vi "solar_ui Resize.vi"(8 "error in (no error)":errorcluster, 9 "Panes":T1={"Status"=TRUE, "Emergency"=TRUE, "Targets"=TRUE}, 10 "MenuRef":refnum<k9>, 11 "VI Refnum":refnum<vi>) -> (0 "error out":errorcluster)   [LabVIEW 2018]
doc: "This resizes the panes of the SOLAR user interface depending on which pane is visible. If the Targets pane is hidden, the emergency stop is hidden as well."
uses:
  <vilib>/Utility/miscctls.llb/LVPointTypeDef.ctl
  solar_ctl SOLAR UI Panes.ctl
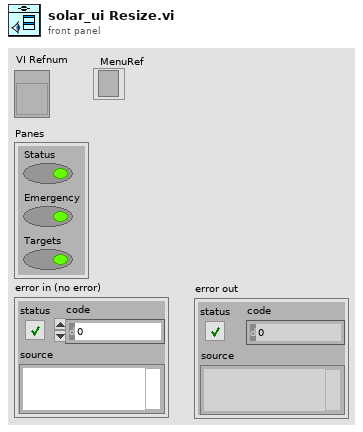
[diagram p1: front panel]
types:
  T1 = typedef "solar_ctl SOLAR UI Panes.ctl" = cluster{"Status":bool, "Emergency":bool, "Targets":bool}
  T2 = enum16{"No Scaling", "Scale All Objects", "Scale Single Object"}
  T3 = typedef "LVBoundsTypeDef.ctl" = cluster{"Width":u32, "Height":u32}
  T4 = typedef "LVMenuShortCut.ctl" = cluster{"include Shift key?":bool, "include Ctrl key?":bool, "shortcut key":string}
  T5 = enum16{"No Scaling", "Scale All Objects", "Scale Single Object"}[]
  T6 = typedef "LVPointTypeDef.ctl" = cluster{"Horizontal":i16, "Vertical":i16}
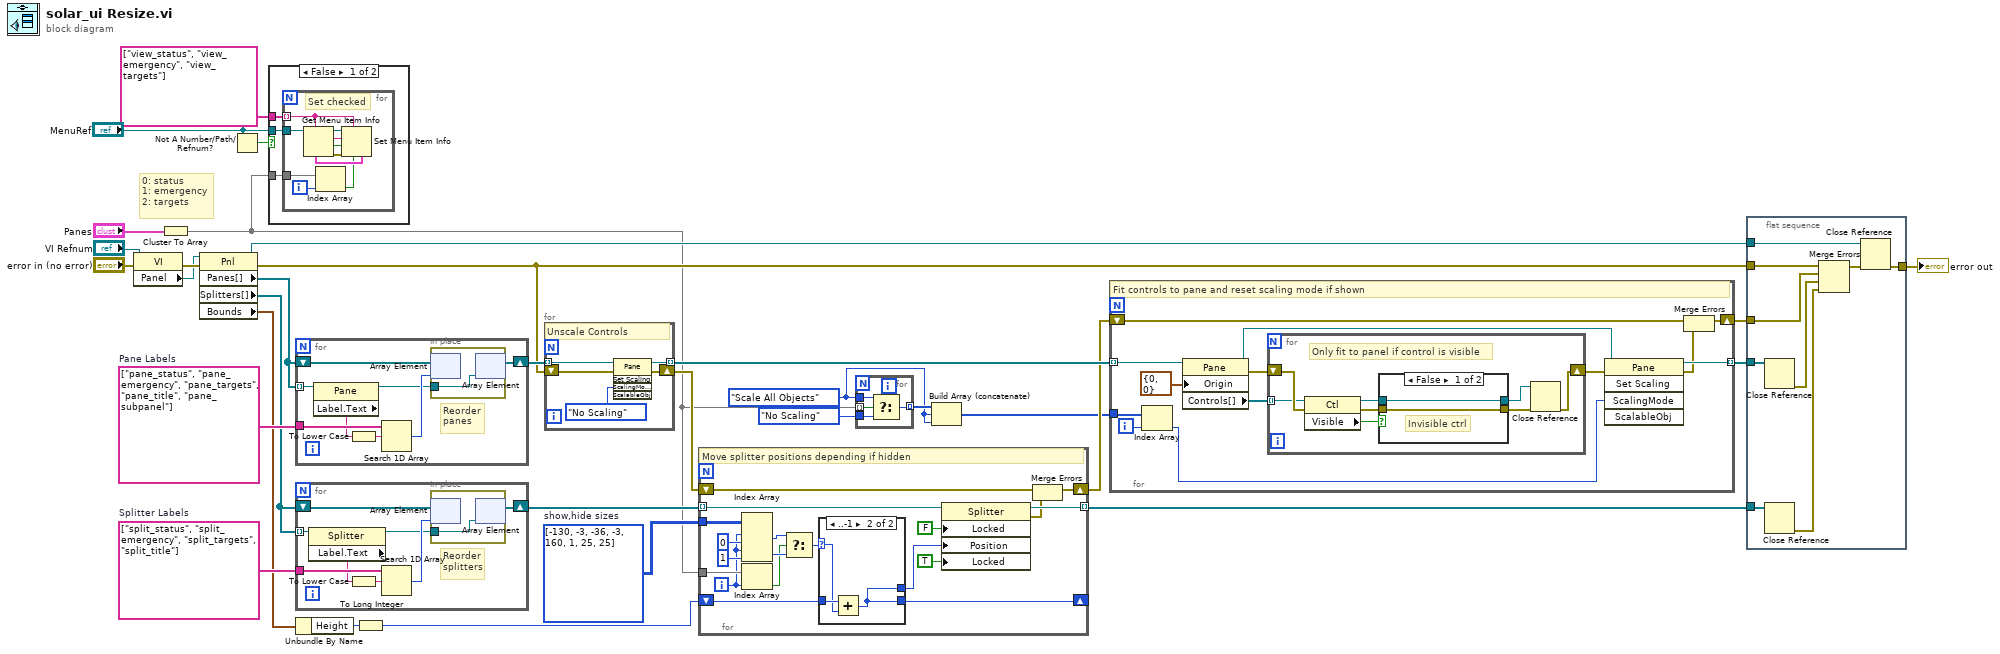
[diagram p0: block diagram]
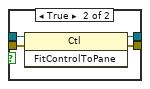
[diagram p3: hidden frame]
diagram:
  w10 = T2."Scale All Objects" ("Scaling Mode")
  w14 = i32[][] [[-130, -3], [-36, -3], [160, 1], [25, 25]]  # show,hide sizes
  w26 = string[] ["split_status", "split_emergency", "split_targets", "split_title"]  # Splitter Labels
  w28 = string[] ["pane_status", "pane_emergency", "pane_targets", "pane_title", "pane_subpanel"]  # Pane Labels
  # "0: status\n1: emergency\n2: targets"
  n1 = property class="VI"(reference="VI Refnum", error in="error in (no error)") -> (error out=w30:errorcluster, "Panel"=w29:refnum<vi>)  [unwired: 1 out]
  n2 = Cluster To Array(cluster="Panes") -> (array=w1:bool[])
  n3 = property class="Pnl"(reference=w29, error in=w30) -> (reference out=w7:refnum<vi>, error out=w21:errorcluster, "Panes[]"=w27:refnum<vi>[], "Splitters[]"=w25:refnum<vi>[], "Bounds"=w3:T3)
  n4 = Not A Number/Path/Refnum?(number/path/refnum="MenuRef") -> (NaN/Path/Refnum?=w4:bool)
  n5 = case shown="False" w4 {
    tunnel: string[] ["view_status", "view_emergency", "view_targets"] -> [w34 _]
    tunnel: "MenuRef" -> [w35 _]
    tunnel: w1 -> [w33 _]
    frame False {
      n6 = for {
        tunnel: w35 -> [w41]
        tunnel: w33 -> [w39]
        tunnel: w34 -> [w36] mode=indexing
        i -> [w38]
        # "Set checked"
        n7 = Get Menu Item Info(7:w36, 11:w41) -> (0:w45:errorcluster, 1:w42:bool, 2:w43:string, 3:w44:refnum<k9>, 6:w40:T4)  [unwired: 1 in, 2 out]
        n8 = Index Array(array=w39, index=w38) -> (element=w37:bool)
        n9 = Set Menu Item Info(4:w40, 6:w37, 7:w36, 8:w45, 9:w42, 10:w43, 11:w44) -> ()  [unwired: 2 out]
      }
    }
    frame True {
    }
  }
  n10 = for {
    tunnel: w27 -> [w53] mode=indexing
    tunnel: w28 -> [w52]
    shift-right: [w46] -> w22
    shift-left: w27 -> [w49]
    # "Reorder\npanes"
    n11 = property class="Pane"(reference=w53) -> (reference out=w47:refnum<vi>, "Label.Text"=w51:string)  [unwired: 1 in, 1 out]
    n12 = To Lower Case(string=w51) -> (all lower case string=w50:string)
    n13 = Search 1D Array(1D array=w52, element=w50) -> (index of element=w48:i32)  [unwired: 1 in]
    n14 = in-place {
      in-place-border: w47 -> [w54]
      n15 = in-place-array #1(w49, w48) -> ()  [unwired: 1 out]
      n16 = in-place-array #1(w54) -> (w46:refnum<vi>[])  [unwired: 1 out]
    }
  }
  n17 = for {
    tunnel: w25 -> [w62] mode=indexing
    tunnel: w26 -> [w61]
    shift-right: [w55] -> w24
    shift-left: w25 -> [w58]
    # "Reorder\nsplitters"
    n18 = property class="Splitter"(reference=w62) -> (reference out=w56:refnum<vi>, "Label.Text"=w60:string)  [unwired: 1 in, 1 out]
    n19 = To Lower Case(string=w60) -> (all lower case string=w59:string)
    n20 = Search 1D Array(1D array=w61, element=w59) -> (index of element=w57:i32)  [unwired: 1 in]
    n21 = in-place {
      in-place-border: w56 -> [w63]
      n22 = in-place-array #2(w58, w57) -> ()  [unwired: 1 out]
      n23 = in-place-array #2(w63) -> (w55:refnum<vi>[])  [unwired: 1 out]
    }
  }
  n24 = Unbundle By Name(w3) -> ("Height"=w13:u32)
  n25 = To Long Integer(number=w13) -> (32bit integer=w8:i32)
  n26 = for {
    tunnel: w22 -> [w68] mode=indexing
    tunnel: [w64] -> w18 mode=indexing
    shift-right: [w65] -> w20
    shift-left: w21 -> [w66]
    # "Unscale Controls"
    n27 = invoke class="Pane" method="Set Scaling"(reference=w68, error in=w66, "ScalingMode"=T2."No Scaling" ("Scaling Mode")) -> (reference out=w64:refnum<vi>, error out=w65:errorcluster)  [unwired: 2 in, 3 out]
  }
  n28 = for {
    tunnel: w24 -> [w87] mode=indexing
    tunnel: [w85] -> w17 mode=indexing
    shift-right: [w72] -> w16
    shift-left: w20 -> [w71]
    tunnel: w14 -> [w83]
    tunnel: w1 -> [w82]
    shift-right: [w77] -> _
    shift-left: w8 -> [w78]
    i -> [w73]
    # "Move splitter positions depending if hidden"
    n29 = Index Array(array=w83, index (row) #1=w73, index (col) #1=0 ("disabled index (col)"), index (row) #2=w73, index (col) #2=1 ("disabled index (col)")) -> (element #1=w80:i32, element #2=w81:i32)
    n30 = Index Array(array=w82, index=w73) -> (element=w74:bool)
    n31 = Select(t=w80, s=w74, f=w81) -> (s? t:f=w79:i32)
    n32 = case shown="..-1" w79 {
      selector: w79 -> [w88 w90]
      tunnel: w78 -> [w89 w92]
      tunnel: [w89 w91] -> w77
      tunnel: [w88 w91] -> w69
      frame 0.. {
      }
      frame ..-1 {
        n33 = Add(x=w92, y=w90) -> (x+y=w91:i32)
      }
    }
    n34 = property class="Splitter"(reference=w87, "Locked"=FALSE ("Splitter Position Locked"), "Position"=w69, "Locked"=TRUE ("Splitter Position Locked")) -> (reference out=w85:refnum<vi>, error out=w70:errorcluster)  [unwired: 1 in]
    n35 = Merge Errors(w71, w70) -> (w72:errorcluster)
  }
  n36 = for {
    tunnel: w1 -> [w96] mode=indexing
    tunnel: w10 -> [w95]
    tunnel: T2."No Scaling" ("Scaling Mode") -> [w94]
    tunnel: [w93] -> w11 mode=indexing
    n37 = Select(t=w95, s=w96, f=w94) -> (s? t:f=w93:T2)
  }
  n38 = Build Array (concatenate)(w11, w10, w10) -> (w9:T5)
  n39 = for {
    tunnel: w18 -> [w109] mode=indexing
    tunnel: [w108] -> w19 mode=indexing
    shift-right: [w104] -> w15
    shift-left: w16 -> [w105]
    tunnel: w9 -> [w106]
    i -> [w107]
    # "Fit controls to pane and reset scaling mode if shown"
    n40 = Index Array(array=w106, index=w107) -> (element=w97:T2)
    n41 = property class="Pane"(reference=w109, "Origin"=T6 {"Horizontal"=0, "Vertical"=0}) -> (reference out=w102:refnum<vi>, error out=w100:errorcluster, "Controls[]"=w98:refnum<vi>[])  [unwired: 1 in]
    n42 = for {
      tunnel: w98 -> [w112] mode=indexing
      shift-right: [w115] -> w99
      shift-left: w100 -> [w117]
      # "Only fit to panel if control is visible"
      n43 = property class="Ctl"(reference=w112, error in=w117) -> (reference out=w111:refnum<vi>, error out=w113:errorcluster, "Visible"=w110:bool)
      n44 = case shown="False" w110 {
        tunnel: [w119 w123] -> w116
        tunnel: [w118 w122] -> w114
        tunnel: w113 -> [w119 w121]
        tunnel: w111 -> [w118 w120]
        frame False {
          # "Invisible ctrl"
        }
        frame True {
          n45 = invoke class="Ctl" method="FitControlToPane"(reference=w120, error in=w121) -> (reference out=w122:refnum<vi>, error out=w123:errorcluster)  [unwired: 1 in, 1 out]
        }
      }
      n46 = Close Reference(reference=w114, error in (no error)=w116) -> (error out=w115:errorcluster)
    }
    n47 = invoke class="Pane" method="Set Scaling"(reference=w102, error in=w99, "ScalingMode"=w97) -> (reference out=w108:refnum<vi>, error out=w103:errorcluster)  [unwired: 2 in, 3 out]
    n48 = Merge Errors(w105, w103) -> (w104:errorcluster)
  }
  n49 = flat-sequence {
    tunnel: [w129] -> w23
    tunnel: w7 -> [w128]
    tunnel: w21 -> [w127]
    tunnel: w19 -> [w126]
    tunnel: w17 -> [w125]
    tunnel: w15 -> [w124]
    frame #0 {
      n50 = Close Reference(reference=w126) -> (error out=w131:errorcluster)  [unwired: 1 in]
      n51 = Close Reference(reference=w125) -> (error out=w130:errorcluster)  [unwired: 1 in]
      n52 = Merge Errors(w127, w124, w131, w130) -> (w132:errorcluster)
      n53 = Close Reference(reference=w128, error in (no error)=w132) -> (error out=w129:errorcluster)
    }
  }
  "error out" <- w23
